vi "Send Query.vi"(8 "error in (no error)":errorcluster, 9 "byte count":u32, 10 "write buffer":string, 11 "VISA resource name":refnum<visa-resource-name>) -> (0 "error out":errorcluster, 2 "read buffer":string, 3 "VISA resource name out":refnum<visa-resource-name>)   [LabVIEW 2023, in "JY-SPEX-TRIAX.lvlib"]
doc: "Sends the given query to the spectrometer and reads back the specified number of bytes."
uses:
  JY-SPEX-TRIAX.lvlib
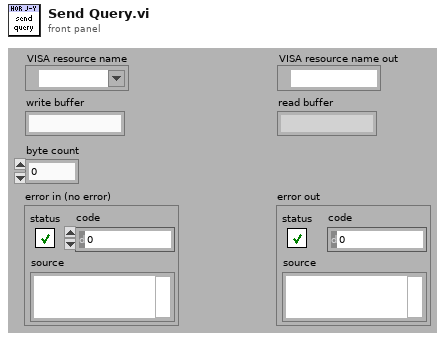
[diagram p1: front panel]
types:
  T1 = typedef "Semaphore RefNum" = refnum<k1>
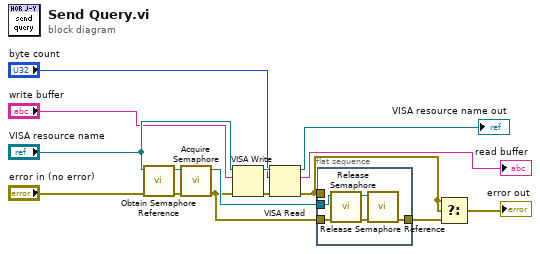
[diagram p0: block diagram]
diagram:
  n1 = call <vilib>:"Obtain Semaphore Reference.vi"("error in (no error)"="error in (no error)", "name (unnamed)"="VISA resource name") -> ("error out"=w15:errorcluster, "semaphore"=w12:T1)  [unwired: 1 in, 3 out]
  n2 = call <vilib>:"Acquire Semaphore.vi"("error in (no error)"=w15, "semaphore"=w12) -> ("error out"=w1:errorcluster, "semaphore out"=w11:T1)  [unwired: 1 in, 3 out]
  n3 = VISA Write(VISA resource name="VISA resource name", write buffer="write buffer", error in (no error)=w1) -> (VISA resource name out=w8:refnum<visa-resource-name>, error out=w9:errorcluster)  [unwired: 1 out]
  n4 = VISA Read(VISA resource name=w8, byte count="byte count", error in (no error)=w9) -> (VISA resource name out=→"VISA resource name out":refnum<visa-resource-name>, read buffer=→"read buffer":string, error out=w4:errorcluster)  [unwired: 1 out]
  n5 = flat-sequence {
    tunnel: w11 -> [w20]
    tunnel: w4 -> [_]
    tunnel: [w17] -> w3
    tunnel: w1 -> [w16]
    frame #0 {
      n6 = call <vilib>:"Release Semaphore.vi"("error in (no error)"=w16, "semaphore"=w20) -> ("error out"=w19:errorcluster, "semaphore out"=w18:T1)  [unwired: 4 out]
      n7 = call <vilib>:"Release Semaphore Reference.vi"("error in (no error)"=w19, "semaphore"=w18) -> ("error out"=w17:errorcluster)  [unwired: 9 out]
    }
  }
  n8 = Select(t=w4, s=w4, f=w3) -> (s? t:f=→"error out":errorcluster)
